vi "ConfigFormatToXMLElement.vi"(9 "Value":string[](array[string]), 10 "Inner Tag":string[](array[string]), 11 "outer Tag":string) -> (3 "Resulting String":string)   [LabVIEW 2018, in "Config.lvlib"]
uses:
  Config.lvlib
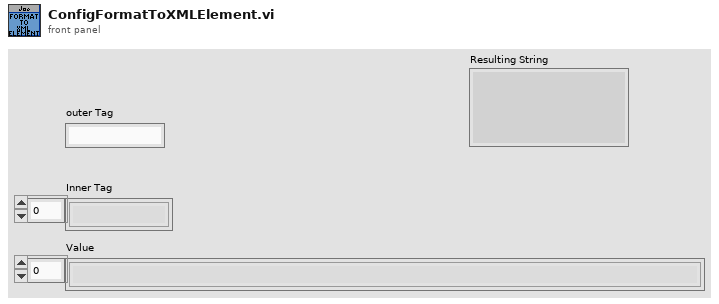
[diagram p1: front panel]
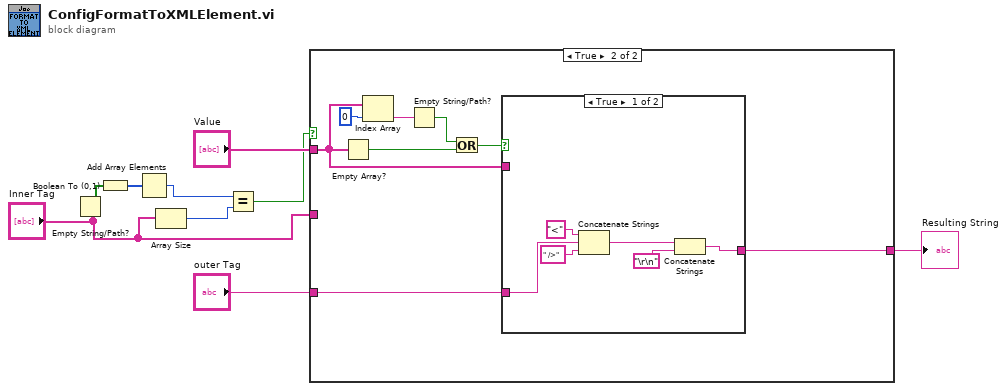
[diagram p0: block diagram]
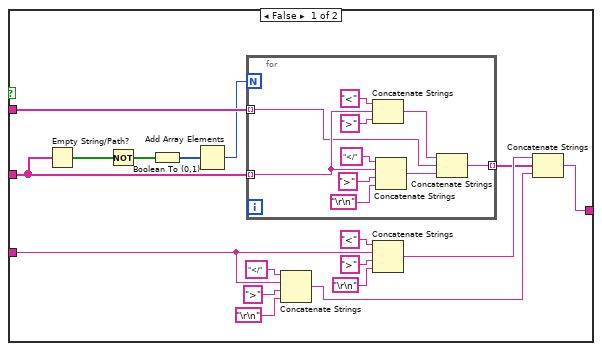
[diagram p2: hidden frame]
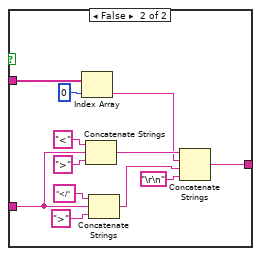
[diagram p3: hidden frame]
diagram:
  n1 = Empty String/Path?(string/path="Inner Tag") -> (empty?=w5:bool[])
  n2 = Boolean To (0,1)(Boolean=w5) -> (0, 1=w6:i16[])
  n3 = Add Array Elements(numeric array=w6) -> (sum=w2:i16)
  n4 = Array Size(array="Inner Tag") -> (size(s)=w3:i32)
  n5 = Equal?(x=w2, y=w3) -> (x = y?=w1:bool)
  n6 = case shown="True" w1 {
    tunnel: "outer Tag" -> [w20 w44]
    tunnel: "Value" -> [w17 w38]
    tunnel: [w15 w43] -> w7
    tunnel: "Inner Tag" -> [w14 _]
    frame False {
      n7 = Empty String/Path?(string/path=w14) -> (empty?=w13:bool[])
      n8 = Not(x=w13) -> (.not. x?=w12:bool[])
      n9 = Boolean To (0,1)(Boolean=w12) -> (0, 1=w10:i16[])
      n10 = Add Array Elements(numeric array=w10) -> (sum=w11:i16)
      n11 = for {
        N: w11 -> [_]
        tunnel: w14 -> [w32] mode=indexing
        tunnel: w17 -> [w29] mode=indexing
        tunnel: [w27] -> w16 mode=indexing
        n12 = Concatenate Strings("<" ("string"), w32, ">" ("string")) -> (w30:string)
        n13 = Concatenate Strings("</" ("string"), w32, ">" ("string"), "\r\n") -> (w28:string)
        n14 = Concatenate Strings(w30, w29, w28) -> (w27:string)
      }
      n15 = Concatenate Strings("</" ("string"), w20, ">" ("string"), "\r\n") -> (w26:string)
      n16 = Concatenate Strings("<" ("string"), w20, ">" ("string"), "\r\n") -> (w25:string)
      n17 = Concatenate Strings(w25, w16, w26) -> (w15:string)
    }
    frame True {
      n18 = Empty Array?(array=w38) -> (empty?=w42:bool)
      n19 = Index Array(array=w38, index=0) -> (element=w37:string)
      n20 = Empty String/Path?(string/path=w37) -> (empty?=w41:bool)
      n21 = Or(x=w41, y=w42) -> (x .or. y?=w40:bool)
      n22 = case shown="True" w40 {
        tunnel: w44 -> [w48 w60]
        tunnel: [w47 w55] -> w43
        tunnel: w38 -> [_ w52]
        frame True {
          n23 = Concatenate Strings("<" ("string"), w48, " />" ("string")) -> (w46:string)
          n24 = Concatenate Strings(w46, "\r\n") -> (w47:string)
        }
        frame False {
          n25 = Index Array(array=w52, index=0) -> (element=w53:string)
          n26 = Concatenate Strings("<" ("string"), w60, ">" ("string")) -> (w57:string)
          n27 = Concatenate Strings("</" ("string"), w60, ">" ("string")) -> (w56:string)
          n28 = Concatenate Strings(w57, w53, w56, "\r\n") -> (w55:string)
        }
      }
    }
  }
  "Resulting String" <- w7
